vi "Write String.vi"(8 "error in":errorcluster, 9 "String":string, 10 "Name":string, 11 "Handle In":i32) -> (0 "error out":errorcluster, 3 "Handle Out":i32, 4 "Error Frame":i32)   [LabVIEW 2024]
panel:
  out "Values Out":dbl[](array[numeric]) format="%.2f"
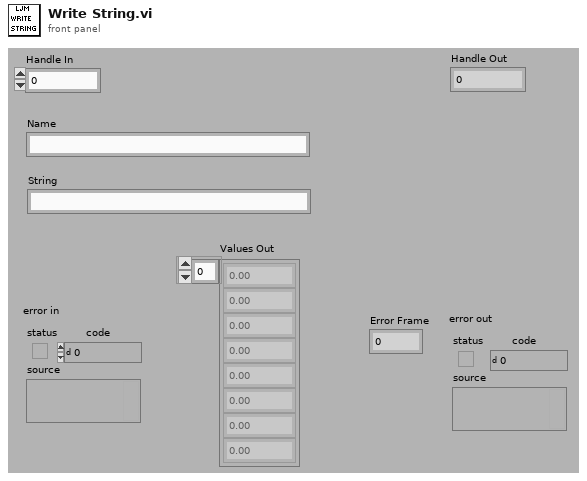
[diagram p1: front panel]
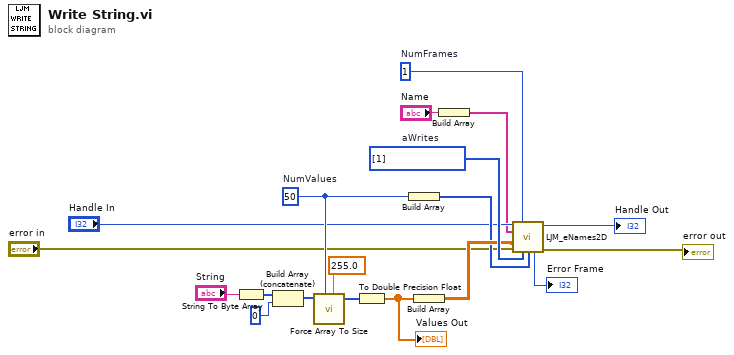
[diagram p0: block diagram]
diagram:
  w8 = 50  # NumValues
  w17 = i32[] [1] items=["Read", "Write"]  # aWrites
  w18 = 1  # NumFrames
  n1 = String To Byte Array(string="String") -> (unsigned byte array=w15:u8[])
  n2 = Build Array (concatenate)(w15, 0) -> (w12:i32[])
  n3 = call "Force Array To Size.vi"("Default Value"=255.0, "# Elements"=w8, "I32 Array In"=w12) -> ("I32 Array Out"=w10:i32[])  [unwired: 4 in, 4 out]
  n4 = To Double Precision Float(number=w10) -> (double precision float=w13:dbl[])
  "Values Out" <- w13
  n5 = Build Array(w8) -> (w9:i32[])
  n6 = Build Array(w13) -> (w16:dbl[][])
  n7 = Build Array("Name") -> (w1:string[])
  n8 = call "LJM_eNames2D.vi"("Handle In"="Handle In", "NumFrames (Auto-Detect)"=w18, "aNames"=w1, "aValuesIn"=w16, "error in"="error in", "aWrites"=w17, "aNumValues"=w9) -> ("Handle Out"=→"Handle Out":i32, "ErrorAddress"=→"Error Frame":i32, "error out"=→"error out":errorcluster)  [unwired: 5 in, 1 out]
